vi "RemoveSpaces.vi"(11 "all rows":string[][](array[string])) -> (3 "Array 2":string[][](array[string]))   [LabVIEW 2023]
uses:
  <vilib>/Utility/file.llb/Read Delimited Spreadsheet (string).vi
panel:
  out "all rows 2":string[][](array[string])
  out "Table Control":string[][](table)
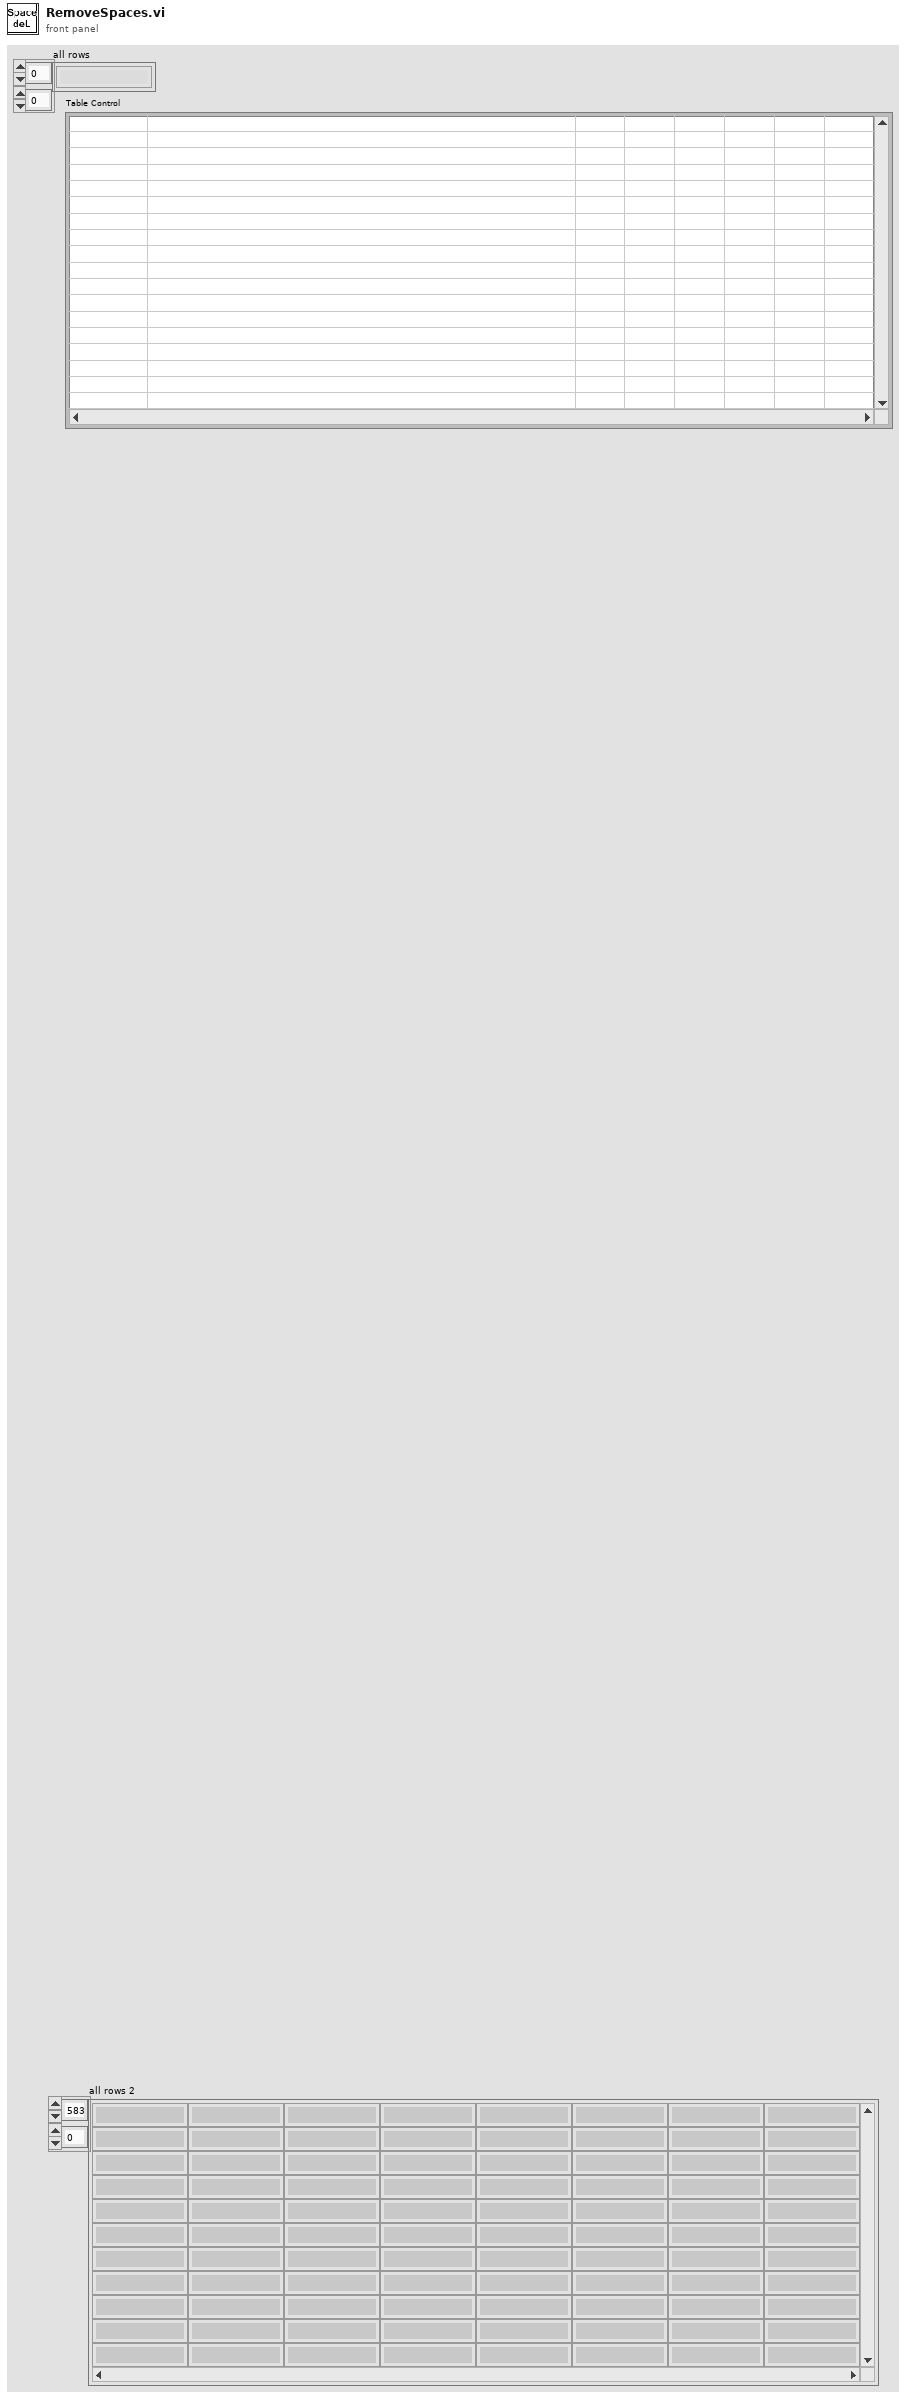
[diagram p1: front panel]
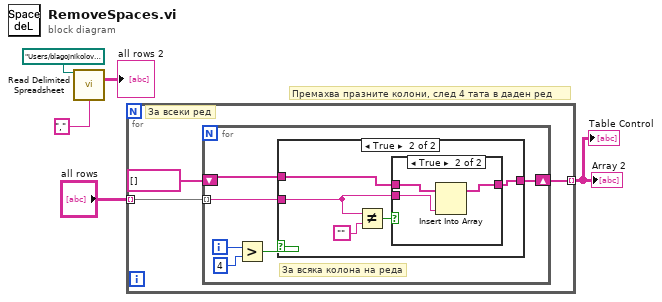
[diagram p0: block diagram]
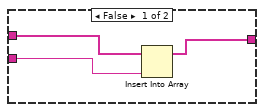
[diagram p2: hidden frame]
diagram:
  # "Премахва празните колони, след 4 тата в даден ред"
  n1 = call-poly <vilib>:"Read Delimited Spreadsheet.vi"("file path (dialog if empty)"=path "/Users/blagojnikolov/Documents/VSCode/report.csv", "delimiter (\\t)"="," ("delimiter (\\t)")) -> ("all rows"=→"all rows 2":string[][])  [unwired: 8 in, 5 out]
  n2 = for {
    tunnel: "all rows" -> [w7] mode=indexing
    tunnel: [w6] -> w2 mode=indexing
    # "За всеки ред"
    n3 = for {
      tunnel: w7 -> [w14] mode=indexing
      shift-right: [w13] -> w6
      shift-left: string[] [] -> [w12]
      i -> [w11]
      # "За всяка колона на реда"
      n4 = Greater?(x=w11, y=4) -> (0:w9:bool)
      n5 = case shown="True" w9 {
        tunnel: w14 -> [w15 w21]
        tunnel: [w16 w20] -> w13
        tunnel: w12 -> [w17 w19]
        frame False {
          n6 = Insert Into Array(array=w17, new element=w15) -> (w16:string[])  [unwired: 1 in]
        }
        frame True {
          n7 = Not Equal?(x=w21, y="") -> (x != y?=w18:bool)
          n8 = case shown="True" w18 {
            tunnel: w21 -> [_ w26]
            tunnel: [w23 w25] -> w20
            tunnel: w19 -> [w23 w24]
            frame False {
            }
            frame True {
              n9 = Insert Into Array(array=w24, new element=w26) -> (w25:string[])  [unwired: 1 in]
            }
          }
        }
      }
    }
  }
  "Array 2" <- w2
  "Table Control" <- w2
